vi "Calculate Shutdown Temperature Change.vi"(9 "Interval":dbl, 10 "Actual Temperature In":dbl, 11 "Required Temperature deg C":dbl) -> (3 "Actual Temperature Out":dbl)   [LabVIEW 2018, in "Thermal Chamber Response Simulator.lvlib"]
doc: "Calculate the change in the temperature based on the specified interval.\n____\nDelacor QMH Thermal Chamber Examples 4.0.0.21\nCopyright (c) 2018, Delacor"
uses:
  Thermal Chamber Response Simulator.lvlib
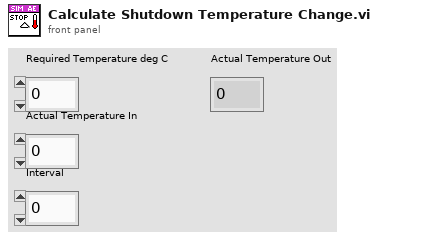
[diagram p1: front panel]
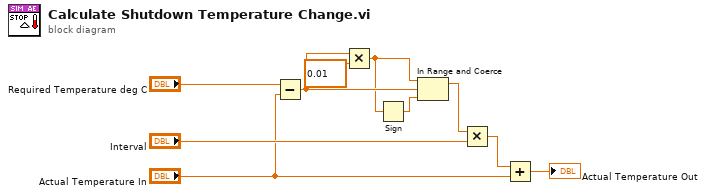
[diagram p0: block diagram]
diagram:
  n1 = Subtract(x="Required Temperature deg C", y="Actual Temperature In") -> (x-y=w3:dbl)
  n2 = Multiply(x=w3, y=0.01 ("Ramp Rate")) -> (x*y=w2:dbl)
  n3 = Sign(1:w2) -> (0:w1:dbl)
  n4 = In Range and Coerce(upper limit=w2, x=w3, lower limit=w1) -> (coerced(x)=w8:dbl)  [unwired: 1 out]
  n5 = Multiply(x=w8, y="Interval") -> (x*y=w9:dbl)
  n6 = Add(x=w9, y="Actual Temperature In") -> (x+y=→"Actual Temperature Out":dbl)
